vi "Record.vi"(8 "error in (no error)":errorcluster, 11 "Spectrum Recorder in":refnum<class "Spectrum Recorder.lvclass">) -> (0 "error out":errorcluster, 3 "Spectrum Recorder out":refnum<class "Spectrum Recorder.lvclass">)   [LabVIEW 2016, in "Spectrum Recorder.lvclass"]
uses:
  Spectrum Recorder.lvclass
  C:/github/LabActor/Worker/Worker.lvclass
  Worker/Worker.lvclass/Worker.ctl
  Spectrum Recorder.lvclass/Spectrum Recorder.ctl
  Template Module/Read State.vi
  NHMFL_Core/Libraries/Red Pitaya/RP Core/RP Transceiver/RP Transceiver.lvclass
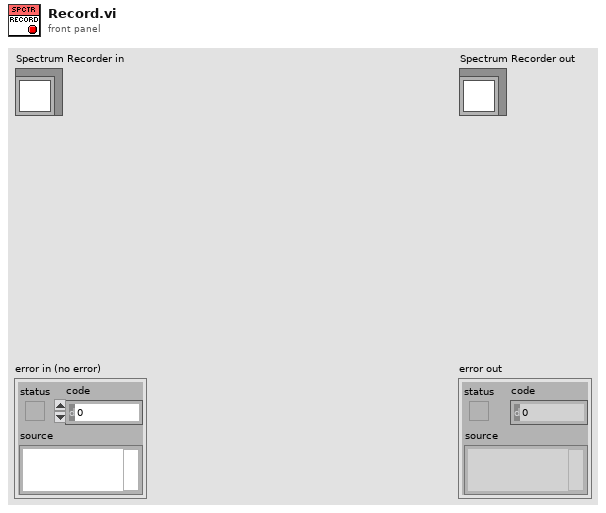
[diagram p1: front panel]
types:
  T1 = typedef "Worker State.ctl" = enum16{"Idle", "Starting", "Working", "Stopping"}
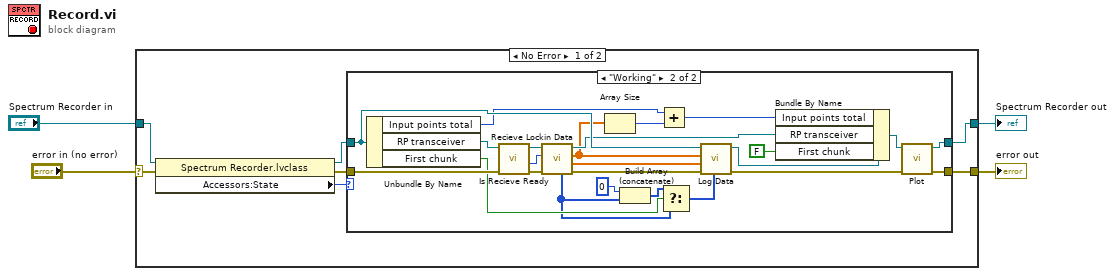
[diagram p0: block diagram]
diagram:
  n1 = case shown="No Error" "error in (no error)" {
    selector: "error in (no error)" -> [w10 w39]
    tunnel: [w9 w39] -> w3
    tunnel: [w11 w38] -> w1
    tunnel: "Spectrum Recorder in" -> [w7 w38]
    frame No Error {
      n2 = property class="Spectrum Recorder.lvclass"(reference=w7, error in=w10) -> (reference out=w6:refnum<class "Spectrum Recorder.lvclass">, error out=w8:errorcluster, "Accessors:State"=w5:T1)
      n3 = case shown="\"Working\"" w5 {
        tunnel: w6 -> [w13 w30]
        tunnel: w8 -> [w12 w36]
        tunnel: [w13 w18] -> w11
        tunnel: [w12 w20] -> w9
        frame "Idle", Default {
        }
        frame "Working" {
          n4 = Unbundle By Name(w30) -> ("Input points total"=w14:i64, "RP transceiver"=w37:refnum<class "RP Transceiver.lvclass">, "First chunk"=w29:bool)
          n5 = call-dynamic "Is Recieve Ready.vi"("error in (no error)"=w36, "RP Instrument in"=w37) -> ("error out"=w35:errorcluster, "Points in buffer"=w33:i32, "RP Instrument out"=w34:refnum<class "RP Transceiver.lvclass">)  [unwired: 6 in, 1 out]
          n6 = call-dynamic "Recieve Lockin Data.vi"("error in (no error)"=w35, "Points to read"=w33, "RP Lockin in"=w34) -> ("error out"=w31:errorcluster, "Volatge X out"=w32:dbl[], "Frequency out"=w17:dbl[], "RP Lockin out"=w23:refnum<class "RP Transceiver.lvclass">, "Starting edges"=w21:i32[])  [unwired: 2 in, 2 out]
          n7 = Array Size(array=w17) -> (size(s)=w15:i32)
          n8 = Build Array (concatenate)(0, w21) -> (w27:i32[])
          n9 = Add(x=w14, y=w15) -> (x+y=w16:i64)
          n10 = Select(t=w27, s=w29, f=w21) -> (s? t:f=w26:i32[])
          n11 = call-dynamic "Log Data.vi"("Edge indexies"=w26, "error in (no error)"=w31, "Volatge"=w32, "Frequency"=w17, "Spectrum Recorder in"=w30) -> ("error out"=w24:errorcluster, "Spectrum Recorder out"=w25:refnum<class "Spectrum Recorder.lvclass">)  [unwired: 5 in]
          n12 = Bundle By Name(cluster=w25, "Input points total"=w16, "RP transceiver"=w23, "First chunk"=FALSE) -> (w19:refnum<class "Spectrum Recorder.lvclass">)
          n13 = call-dynamic "Plot.vi"("error in (no error)"=w24, "Spectrum Recorder in"=w19) -> ("error out"=w20:errorcluster, "Spectrum Recorder out"=w18:refnum<class "Spectrum Recorder.lvclass">)  [unwired: 8 in]
        }
      }
    }
    frame Error {
    }
  }
  "error out" <- w3
  "Spectrum Recorder out" <- w1
